vi "condAmbientalesIniciales.vi"(8 "error in (no error)":errorcluster, 11 "Calibrador in":refnum<class "Calibrador.lvclass">) -> (0 "error out":errorcluster, 3 "Calibrador out":refnum<class "Calibrador.lvclass">)   [LabVIEW 2019, in "Calibrador.lvclass"]
uses:
  Calibrador.lvclass
  Base de Datos/SQLiteConnector/SQLiteConnection.lvclass
  Base de Datos/Base de Datos.lvclass
panel:
  in  "salir":bool
  in  "presion":dbl
  out "presion_corregida":dbl
  out "presion_ok":bool
  in  "humedad":dbl
  out "humedad_corregida":dbl
  out "humedad_ok":bool
  in  "temperatura":dbl
  out "temp_corregida":dbl
  out "temp_ok":bool
  # "Medido"
  # "Corregido"
  # "Cumple"
  # "[°C]"
  # "[hPa]"
  # "[%]"
  # "Humedad"
  # "Presión"
  # "Temperatura"
  # "Condiciones Ambientales \nINICIALES"
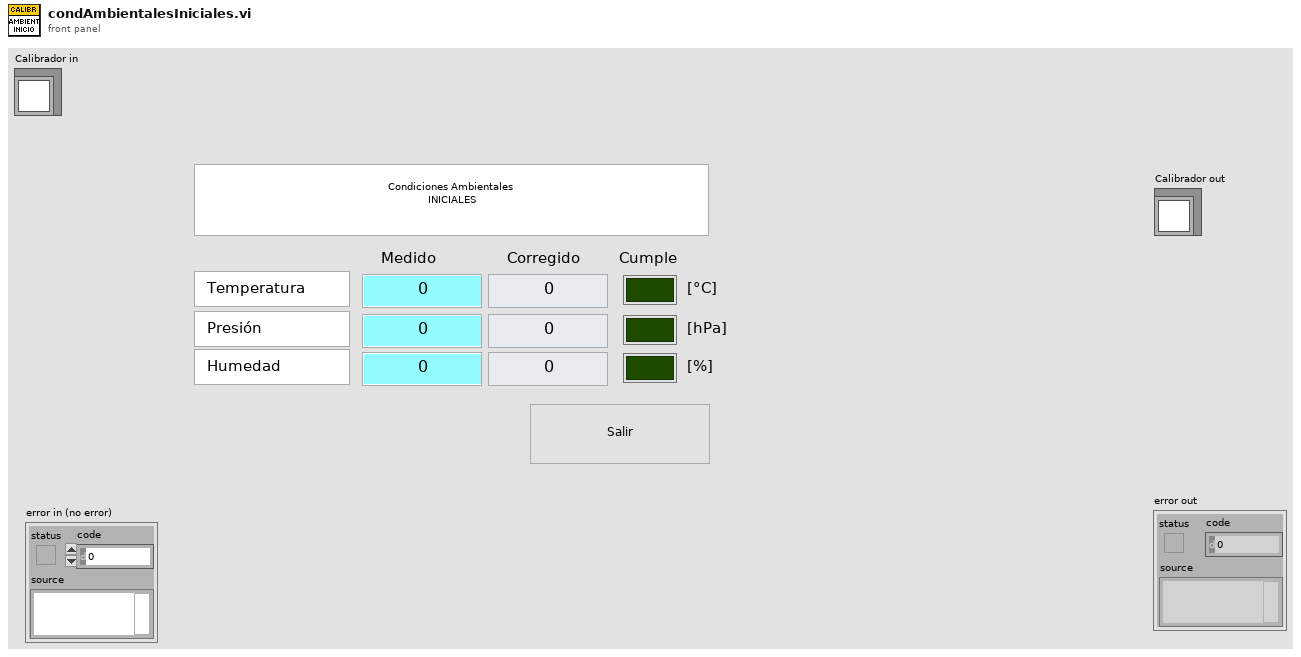
[diagram p1: front panel]
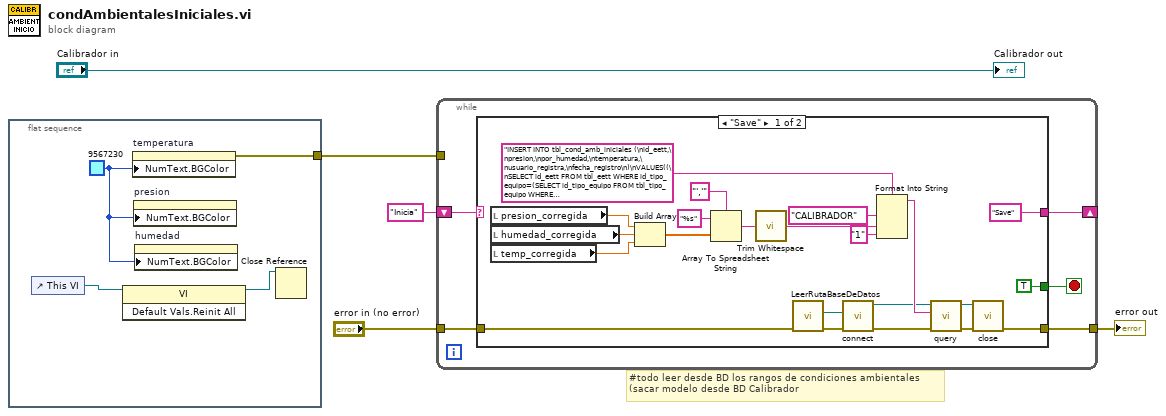
[diagram p0: block diagram]
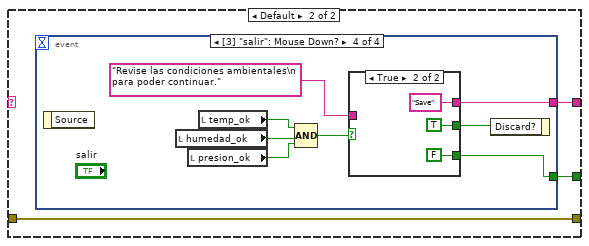
[diagram p2: hidden frame]
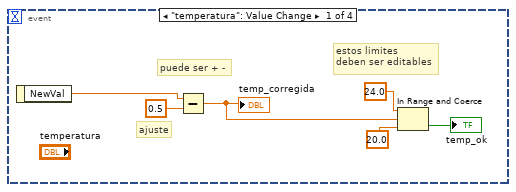
[diagram p3: hidden frame]
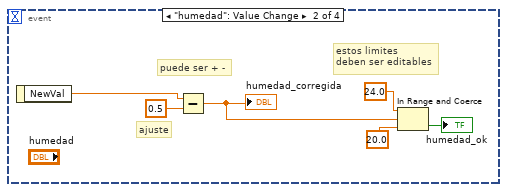
[diagram p4: hidden frame]
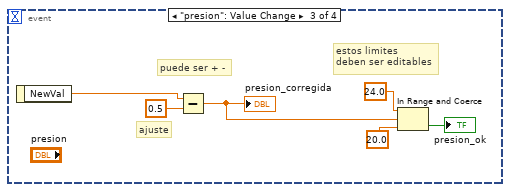
[diagram p5: hidden frame]
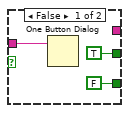
[diagram p6: hidden frame]
diagram:
  # "#todo leer desde BD los rangos de condiciones ambientales\n(sacar modelo desde BD Calibrador"
  n1 = flat-sequence {
    tunnel: [w8] -> w4
    frame #0 {
      w9 = u32 9567230
      n2 = control-ref of="This VI"() -> (w7:refnum<vi>)
      n3 = invoke class="VI" method="Default Vals.Reinit All"(reference=w7) -> (reference out=w6:refnum<vi>)  [unwired: 2 in, 2 out]
      n4 = property on="temperatura" class="DigNum (strict)"("NumText.BGColor"=w9) -> (error out=w8:errorcluster)  [unwired: 2 in, 1 out]
      n5 = property on="presion" class="DigNum (strict)"("NumText.BGColor"=w9) -> ()  [unwired: 2 in, 2 out]
      n6 = property on="humedad" class="DigNum (strict)"("NumText.BGColor"=w9) -> ()  [unwired: 2 in, 2 out]
      n7 = Close Reference(reference=w6) -> ()  [unwired: 1 in, 1 out]
    }
  }
  n8 = while {
    tunnel: w4 -> [_]
    shift-right: [w12] -> _
    shift-left: "Inicia" -> [w13]
    tunnel: "error in (no error)" -> [w11]
    tunnel: [w10] -> w1
    stop <- w14 stop-if-true
    n9 = case shown="\"Save\"" w13 {
      tunnel: [TRUE w39] -> w14
      tunnel: ["Save" w38] -> w12
      tunnel: w11 -> [w16 w37]
      tunnel: [w15 w37] -> w10
      frame "Save" {
        n10 = local read "presion_corregida"() -> (w18:dbl)
        n11 = local read "humedad_corregida"() -> (w19:dbl)
        n12 = local read "temp_corregida"() -> (w17:dbl)
        n13 = Build Array(w18, w19, w17) -> (w29:dbl[])
        n14 = Array To Spreadsheet String(delimiter (Tab)="','", array=w29, 3:"%s" ("format string")) -> (spreadsheet string=w33:string)
        n15 = call <vilib>:"Trim Whitespace.vi"("string"=w33) -> ("trimmed string"=w34:string)  [unwired: 1 in]
        n16 = call "LeerRutaBaseDeDatos.vi"("error in (no error)"=w16) -> ("error out"=w26:errorcluster, "Database Path"=w25:path)  [unwired: 9 in]
        n17 = call "connect.vi"("error in (no error)"=w26, "Database Path"=w25) -> ("error out"=w23:errorcluster, "object out"=w24:refnum<class "SQLiteConnection.lvclass">)  [unwired: 8 in]
        n18 = Format Into String(format string="INSERT INTO tbl_cond_amb_iniciales (\nid_eett,\npresion,\npor_humedad,\ntemperatura,\nusuario_registra,\nfecha_registro\n)\nVALUES((\nSELECT id_eett FROM tbl_eett WHERE id_tipo_equipo=(SELECT id_tipo_equipo FROM tbl_tipo_equipo WHERE nombre='%s')),'%s','%s',DATETIME('NOW'))" ("SQL Statement"), "CALIBRADOR" ("input 1"), w34, "1" ("input 2")) -> (resulting string=w28:string)  [unwired: 2 in, 1 out]
        n19 = call "query.vi"("error in (no error)"=w23, "SQL Statement"=w28, "object in"=w24) -> ("error out"=w21:errorcluster, "object out"=w22:refnum<class "SQLiteConnection.lvclass">)  [unwired: 5 in, 2 out]
        n20 = call-dynamic "close.vi"("error in (no error)"=w21, "object in"=w22) -> ("error out"=w15:errorcluster)  [unwired: 8 in, 1 out]
      }
      frame Default {
        n21 = event shown="[3] \"salir\": Mouse Down?" {
          selector: _ -> [_ _ _ _]
          dyn-events: _ -> [_ _ _ _]
          timeout: _ -> [_ _ _ _]
          tunnel: [_ _ _ w59] -> w39
          tunnel: [_ _ _ w58] -> w38
          event "temperatura": Value Change {
            # "estos limites\ndeben ser editables"
            # "puede ser + -"
            # "ajuste"
            n22 = event-data() -> ("NewVal"=w40:dbl)  [unwired: 1 in]
            n23 = Subtract(x=w40, y=0.5) -> (x-y=w45:dbl)
            "temp_corregida" <- w45
            n24 = In Range and Coerce(upper limit=24.0, x=w45, lower limit=20.0) -> (In Range?=→"temp_ok":bool)  [unwired: 1 out]
          }
          event "humedad": Value Change {
            # "estos limites\ndeben ser editables"
            # "puede ser + -"
            # "ajuste"
            n25 = event-data() -> ("NewVal"=w48:dbl)  [unwired: 1 in]
            n26 = Subtract(x=w48, y=0.5) -> (x-y=w47:dbl)
            "humedad_corregida" <- w47
            n27 = In Range and Coerce(upper limit=24.0, x=w47, lower limit=20.0) -> (In Range?=→"humedad_ok":bool)  [unwired: 1 out]
          }
          event "presion": Value Change {
            # "estos limites\ndeben ser editables"
            # "puede ser + -"
            # "ajuste"
            n28 = event-data() -> ("NewVal"=w54:dbl)  [unwired: 1 in]
            n29 = Subtract(x=w54, y=0.5) -> (x-y=w53:dbl)
            "presion_corregida" <- w53
            n30 = In Range and Coerce(upper limit=24.0, x=w53, lower limit=20.0) -> (In Range?=→"presion_ok":bool)  [unwired: 1 out]
          }
          event "salir": Mouse Down? {
            n31 = event-data() -> ()  [unwired: 1 in, 1 out]
            n32 = local read "humedad_ok"() -> (w64:bool)
            n33 = local read "presion_ok"() -> (w63:bool)
            n34 = local read "temp_ok"() -> (w65:bool)
            n35 = Compound Arithmetic op=AND(w65, w64, w63) -> (w62:bool)
            n36 = case shown="True" w62 {
              tunnel: "Revise las condiciones ambientales\n           para poder continuar." -> [w68 _]
              tunnel: [TRUE TRUE] -> w60
              tunnel: [FALSE FALSE] -> w59
              tunnel: [_ "Save"] -> w58
              frame False {
                n37 = One Button Dialog(message=w68) -> ()  [unwired: 1 in, 1 out]
              }
              frame True {
              }
            }
            n38 = event-data("Discard?"=w60) -> ()  [unwired: 1 in, 1 out]
          }
        }
      }
    }
  }
  "error out" <- w1
  "Calibrador out" <- "Calibrador in"
